vi "K-Vector.vi"(10 "i-th word":i32, 11 "Round":i32) -> (2 "k":i32)   [LabVIEW 2013, in "MD5.lvlib" / "MD5.lvclass"]
uses:
  MD5.lvclass
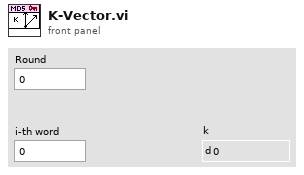
[diagram p1: front panel]
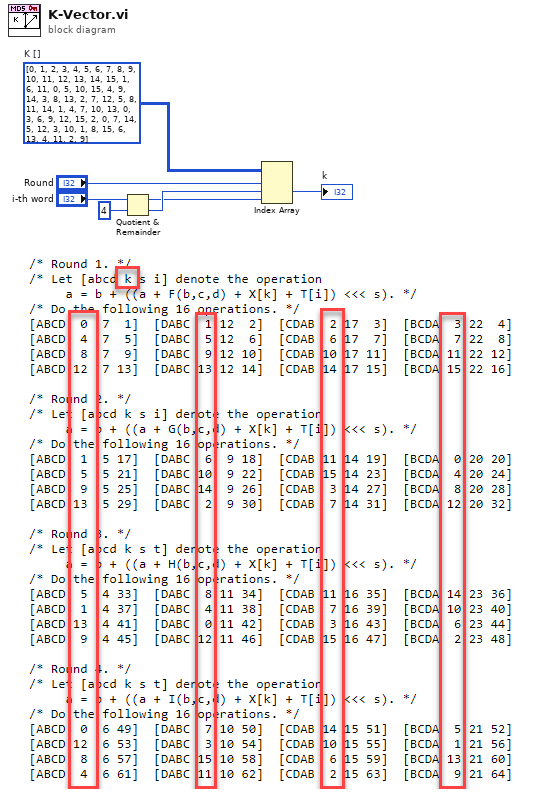
[diagram p0: block diagram]
diagram:
  w6 = i32[][][] [[[0, 1, 2, 3], [4, 5, 6, 7], [8, 9, 10, 11], [12, 13, 14, 15]], [[1, 6, 11, 0], [5, 10, 15, 4], [9, 14, 3, 8], [13, 2, 7, 12]], [[5, 8, 11, 14], [1, 4, 7, 10], [13, 0, 3, 6], [9, 12, 15, 2]], [[0, 7, 14, 5], [12, 3, 10, 1], [8, 15, 6, 13], [4, 11, 2, 9]]]  # K []
  n1 = Quotient & Remainder(x="i-th word", y=4) -> (x-y*floor(x/y)=w3:i32, floor(x/y)=w4:i32)
  n2 = Index Array(array=w6, index (dim 0)="Round", index (dim 1)=w4, index (dim 2)=w3) -> (element=→"k":i32)
